vi "find accelerometer to calibrate.vi"(0 "All Files in Dir":path[](array[path]), 1 "Frecuencia de muestreo (Hz)":dbl, 2 "Pattern frequency (Hz)":dbl, 3 "Calibration":T1, 4 "Elementos":i32) -> (7 "Calibration out":T1, 8 "Data":sgl[][][](array[numeric]), 9 "1 accel found?":bool[](array[boolean]))   [LabVIEW 2015]
doc: "If there is only one accelerometer connected returns the index it is in"
uses:
  controls/Calibration Data.ctl
  <vilib>/Analysis/5stat.llb/RMS (DBL).vi
  <vilib>/measure/madcrms.llb/Basic Averaged DC-RMS for 1 Chan.vi
  <vilib>/measure/NI_MAPro.lvlib
  <vilib>/Analysis/NI_AALPro.lvlib
panel:
  out "size(s) 3":i32
  out "size(s)":i32[](array[numeric])
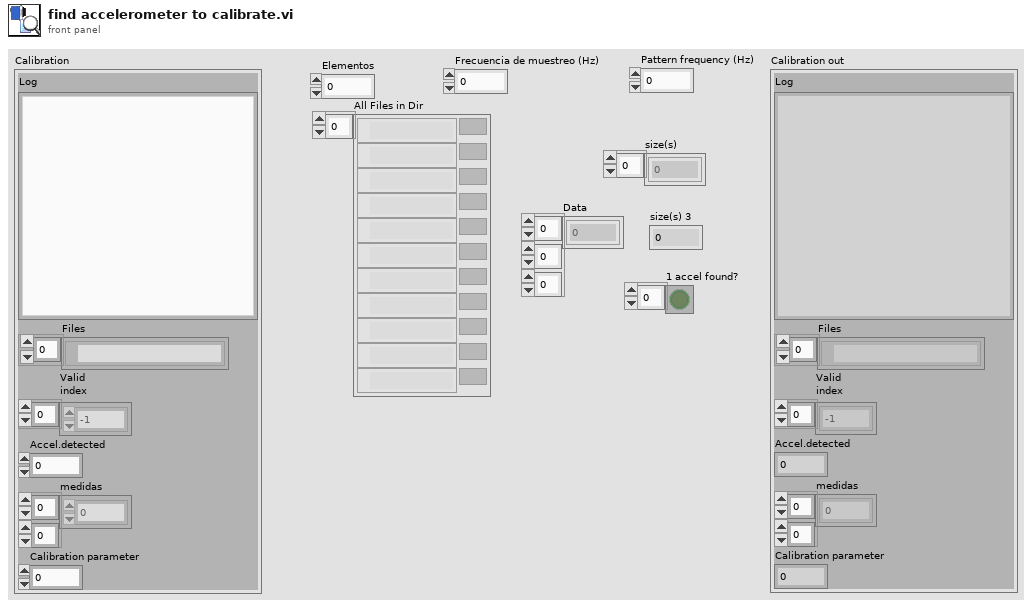
[diagram p1: front panel]
types:
  T1 = typedef "Calibration Data.ctl" = cluster{"Log":string, "Files":path[], "Valid\nindex":i32[], "Accel.detected":i32, "medidas":sgl[][], "Calibration parameter":dbl}
  T2 = enum16{"big-endian, network order", "native, host order", "little-endian"}
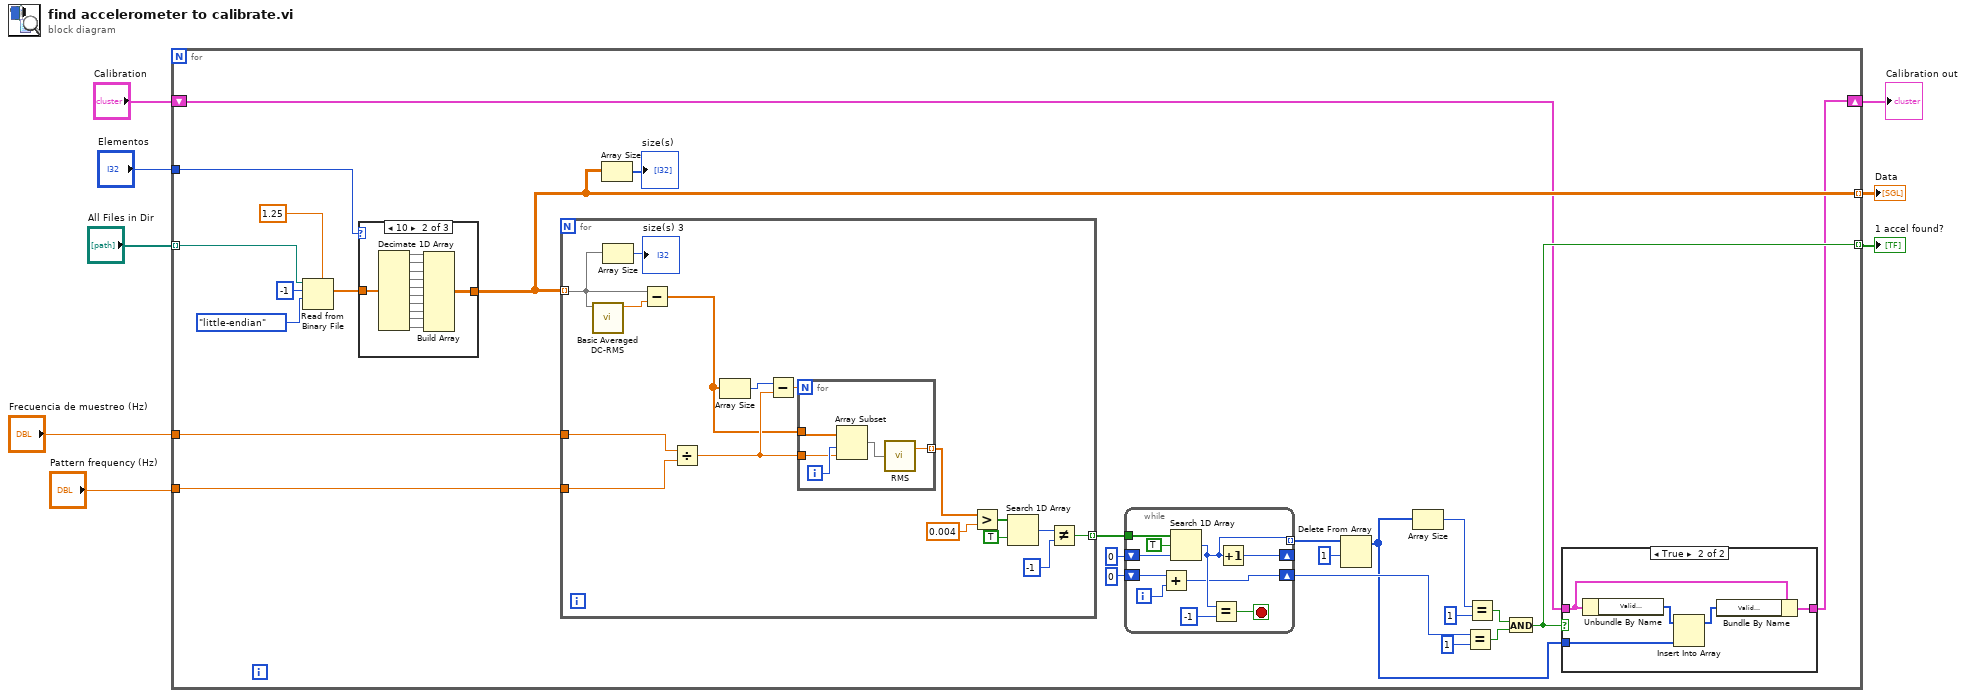
[diagram p0: block diagram]
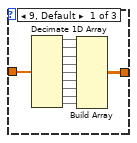
[diagram p3: hidden frame]
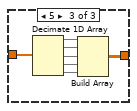
[diagram p4: hidden frame]
diagram:
  n1 = for {
    tunnel: "All Files in Dir" -> [w29] mode=indexing
    tunnel: [w11] -> w1 mode=indexing
    tunnel: [w13] -> w3 mode=indexing
    tunnel: "Elementos" -> [w18]
    tunnel: "Frecuencia de muestreo (Hz)" -> [w17]
    tunnel: "Pattern frequency (Hz)" -> [w16]
    shift-right: [w9] -> w2
    shift-left: "Calibration" -> [w10]
    n2 = Read from Binary File(5:sgl 1.25, 9:T2."little-endian" ("byte order (0:big-endian, network order)"), 10:-1 ("count (1)"), 11:w29) -> (2:w30:sgl[])  [unwired: 1 in, 4 out]
    n3 = case shown="10" w18 {
      tunnel: [w50 w63 w73] -> w13
      tunnel: w30 -> [w51 w61 w74]
      frame 9, Default {
        n4 = Decimate 1D Array(w51) -> (w52:sgl[], w60:sgl[], w59:sgl[], w55:sgl[], w54:sgl[], w56:sgl[], w57:sgl[], w58:sgl[], w53:sgl[])
        n5 = Build Array(w52, w60, w59, w55, w54, w56, w57, w58, w53) -> (w50:sgl[][])
      }
      frame 10 {
        n6 = Decimate 1D Array(w61) -> (w62:sgl[], w72:sgl[], w71:sgl[], w67:sgl[], w66:sgl[], w68:sgl[], w69:sgl[], w70:sgl[], w65:sgl[], w64:sgl[])
        n7 = Build Array(w62, w72, w71, w67, w66, w68, w69, w70, w65, w64) -> (w63:sgl[][])
      }
      frame 5 {
        n8 = Decimate 1D Array(w74) -> (w75:sgl[], w79:sgl[], w78:sgl[], w77:sgl[], w76:sgl[])
        n9 = Build Array(w75, w79, w78, w77, w76) -> (w73:sgl[][])
      }
    }
    n10 = for {
      tunnel: w13 -> [w82] mode=indexing
      tunnel: [w85] -> w26 mode=indexing
      tunnel: w17 -> [w84]
      tunnel: w16 -> [w83]
      n11 = call-poly <vilib>:"Basic Averaged DC-RMS.vi"("signal in"=w82) -> ("DC value"=w95:dbl)  [unwired: 7 in, 3 out]
      n12 = Array Size(array=w82) -> (size(s)=→"size(s) 3":i32)
      n13 = Subtract(x=w82, y=w95) -> (x-y=w91:dbl[])
      n14 = Divide(x=w84, y=w83) -> (x/y=w92:dbl)
      n15 = Array Size(array=w91) -> (size(s)=w93:i32)
      n16 = Subtract(x=w93, y=w92) -> (x-y=w94:dbl)
      n17 = for {
        N: w94 -> [_]
        tunnel: w92 -> [w97]
        tunnel: [w100] -> w80 mode=indexing
        tunnel: w91 -> [w99]
        i -> [w98]
        n18 = Array Subset(array=w99, index=w98, length=w97) -> (w96:dbl[])
        n19 = call-poly <vilib>:"RMS.vi"("X"=w96) -> ("rms value"=w100:dbl)  [unwired: 1 out]
      }
      n20 = Greater?(x=w80, y=0.004 ("threshold y")) -> (0:w89:bool[])
      n21 = Search 1D Array(1D array=w89, element=TRUE) -> (index of element=w87:i32)  [unwired: 1 in]
      n22 = Not Equal?(x=w87, y=-1) -> (x != y?=w85:bool)
    }
    n23 = Array Size(array=w13) -> (size(s)=→"size(s)":i32[])
    n24 = while {
      tunnel: w26 -> [w49]
      shift-right: [w42] -> _
      shift-left: 0 ("index of element") -> [w46]
      shift-right: [w40] -> w19
      shift-left: 0 ("index of element") -> [w43]
      tunnel: [w41] -> w15 mode=indexing
      i -> [w44]
      stop <- w47 stop-if-true
      n25 = Add(x=w43, y=w44) -> (x+y=w40:i32)
      n26 = Search 1D Array(1D array=w49, element=TRUE, start index (0)=w46) -> (index of element=w41:i32)
      n27 = Equal?(x=w41, y=-1) -> (x = y?=w47:bool)
      n28 = Increment(x=w41) -> (x+1=w42:i32)
    }
    n29 = Delete From Array(array=w15, length=1) -> (array with subset deleted=w14:i32[])  [unwired: 1 in, 1 out]
    n30 = Array Size(array=w14) -> (size(s)=w22:i32)
    n31 = Equal?(x=w19, y=1) -> (x = y?=w21:bool)
    n32 = Equal?(x=w22, y=1) -> (x = y?=w20:bool)
    n33 = And(x=w20, y=w21) -> (x .and. y?=w11:bool)
    n34 = case shown="True" w11 {
      tunnel: w14 -> [_ w39]
      tunnel: w10 -> [w34 w36]
      tunnel: [w34 w35] -> w9
      frame False {
      }
      frame True {
        n35 = Unbundle By Name(w36) -> ("Valid\nindex"=w38:i32[])
        n36 = Insert Into Array(array=w38, new element=w39) -> (w37:i32[])  [unwired: 1 in]
        n37 = Bundle By Name(cluster=w36, "Valid\nindex"=w37) -> (w35:T1)
      }
    }
  }
  "Calibration out" <- w2
  "Data" <- w3
  "1 accel found?" <- w1
